vi "Clear.vi"(8 "error in (no error)":errorcluster, 11 "Test Tree In":refnum<class "Test Tree.lvclass">) -> (0 "error out":errorcluster)   [LabVIEW 2020, in "Test Tree.lvclass"]
uses:
  Test Tree.lvclass
  Test Tree.lvclass/Test Tree.ctl
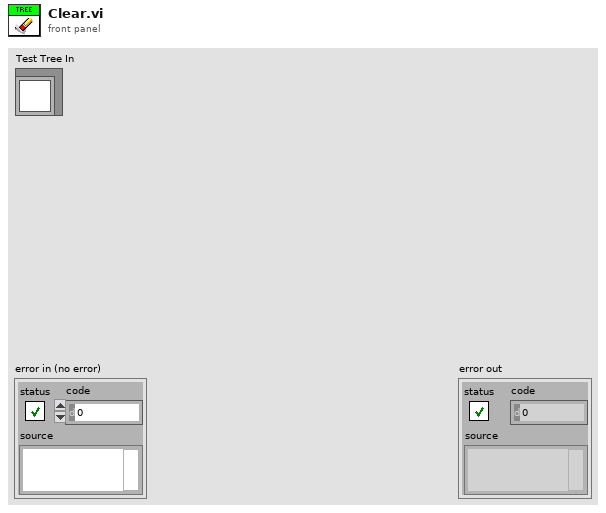
[diagram p1: front panel]
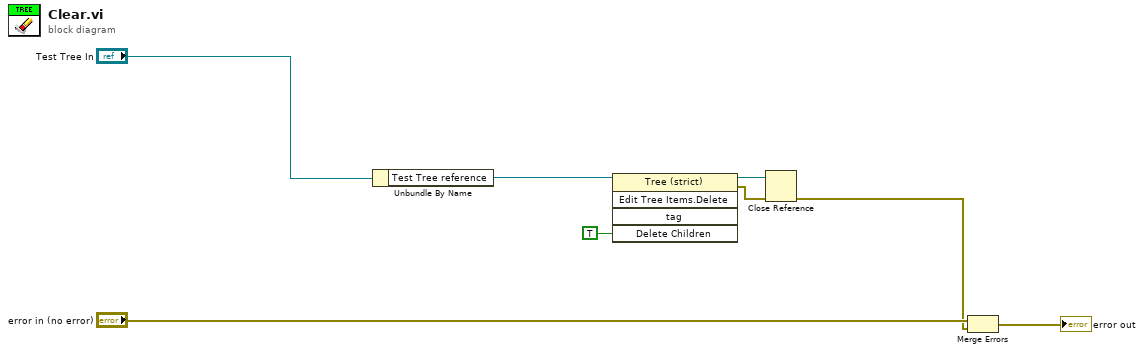
[diagram p0: block diagram]
diagram:
  n1 = Unbundle By Name("Test Tree In") -> ("Test Tree reference"=w3:refnum<vi>)
  n2 = invoke on="Invoke Node" class="Tree (strict)" method="Edit Tree Items.Delete"(reference=w3, "Delete Children"=TRUE ("Delete Children?")) -> (reference out=w2:refnum<vi>, error out=w1:errorcluster)  [unwired: 3 in, 3 out]
  n3 = Close Reference(reference=w2, error in (no error)=w1) -> (error out=w5:errorcluster)
  n4 = Merge Errors("error in (no error)", w5) -> (→"error out":errorcluster)
